vi "singleTrial_noReturn_TRAINING.vi"() -> ()   [LabVIEW 2017]
uses:
  <vilib>/Utility/file.llb/Read Delimited Spreadsheet (DBL).vi
  <vilib>/Utility/file.llb/Write Delimited Spreadsheet (I64).vi
panel:
  in  "difficulty":string(combo)="1"
  in  "Maze rotation":string(combo)="clockwise"
  in  "Choice/goal platforms up or down?":string(combo)="up"
  in  "Rat ID":string
  out "choices":i32[][](array[numeric])
  in  "Goal \nplatform":i32
  in  "start platform":i32
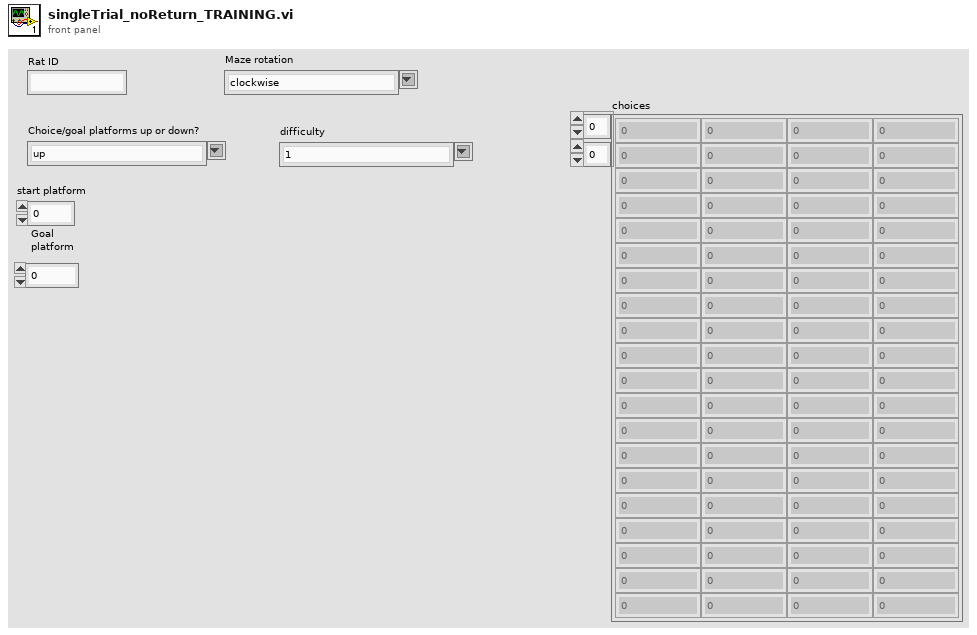
[diagram p1: front panel]
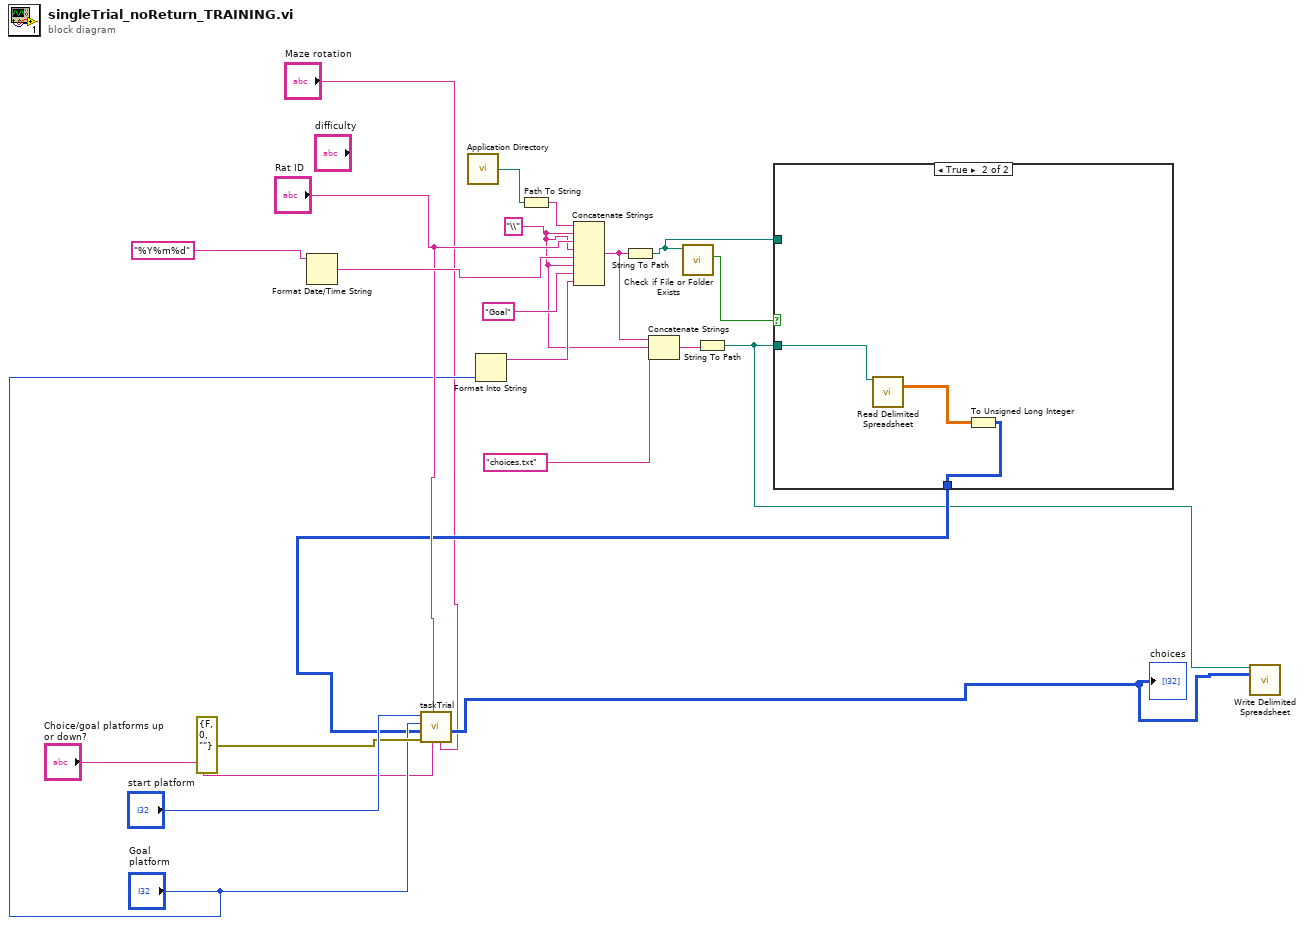
[diagram p0: block diagram]
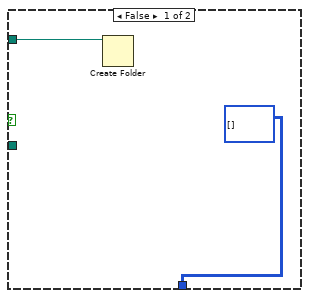
[diagram p2: hidden frame]
diagram:
  w10 = "\\" ("string")
  n1 = Format Date/Time String(time format string (%c)="%Y%m%d" ("time string")) -> (date/time string=w17:string)  [unwired: 2 in]
  n2 = call <vilib>:"Application Directory.vi"() -> ("Application Directory"=w16:path)
  n3 = Format Into String("Goal \nplatform") -> (resulting string=w12:string)  [unwired: 3 in, 1 out]
  n4 = Path To String(path=w16) -> (string=w19:string)
  n5 = Concatenate Strings(w19, w10, "Rat ID", w10, w17, w10, "Goal" ("string"), w12) -> (w9:string)
  n6 = String To Path(string=w9) -> (path=w5:path)
  n7 = Concatenate Strings(w9, w10, "choices.txt" ("string")) -> (w7:string)
  n8 = call <vilib>:"Check if File or Folder Exists.vi"("path"=w5) -> ("file or folder exists?"=w11:bool)  [unwired: 8 in, 2 out]
  n9 = String To Path(string=w7) -> (path=w4:path)
  n10 = case shown="True" w11 {
    tunnel: w4 -> [_ w26]
    tunnel: [i32[][] [] ("previousChoices") w24] -> w6
    tunnel: w5 -> [w22 _]
    frame False {
      n11 = Create Folder(path (use dialog)=w22) -> ()  [unwired: 2 in, 3 out]
    }
    frame True {
      n12 = call-poly <vilib>:"Read Delimited Spreadsheet.vi"("file path (dialog if empty)"=w26) -> ("all rows"=w25:dbl[][])  [unwired: 9 in, 5 out]
      n13 = To Unsigned Long Integer(number=w25) -> (unsigned 32bit integer=w24:u32[][])
    }
  }
  n14 = call "taskTrial.vi"("mazeDirection"="Maze rotation", "up or down"="Choice/goal platforms up or down?", "Rat ID"="Rat ID", "error in (no error)"=errorcluster {"status"=FALSE, "code"=0, "source"=""}, "previousChoices"=w6, "Goal \nplatform"="Goal \nplatform", "Start \nplatform"="start platform") -> ("previousChoices updated"=w2:i32[][])  [unwired: 2 in, 2 out]
  "choices" <- w2
  n15 = call-poly <vilib>:"Write Delimited Spreadsheet.vi"("file path (dialog if empty)"=w4, "2D data"=w2) -> ()  [unwired: 12 in, 2 out]
